vi "ParamReader2.vi"(8 "error in (no error)":errorcluster, 10 "what kind of binary":i32, 11 "selected path":path caption="selected \"*.par\" path") -> (0 "error out":errorcluster, 2 "CodeString":string, 5 "Cluster":T1 {"AdcOffset" format="%#.6f"; "AdcScale" format="%#.6f"})   [LabVIEW 2014]
panel:
  out "slow ADC\nactiveChannels\nRange":string
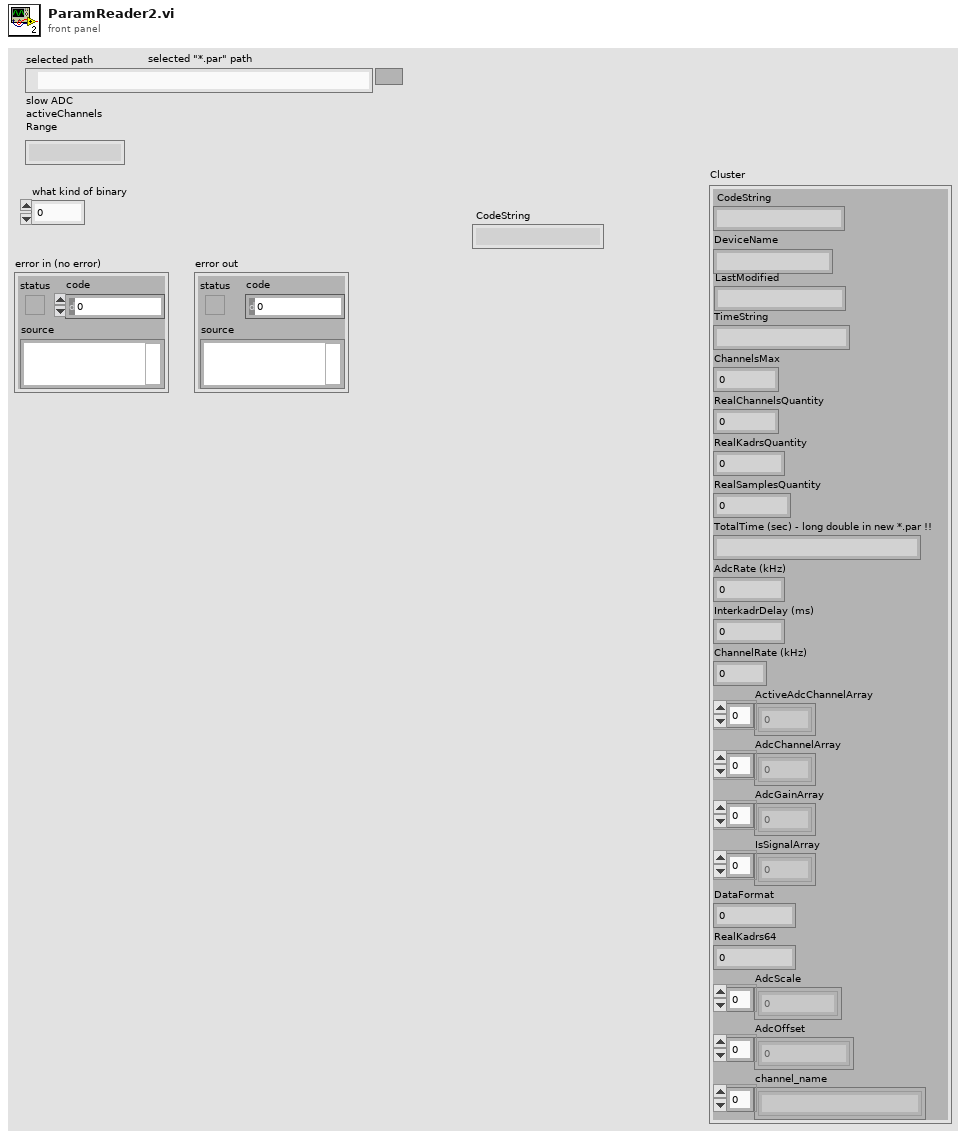
[diagram p1: front panel]
types:
  T1 = cluster{" CodeString":string, "DeviceName":string, "TimeString":string, "ChannelsMax":i16, "RealChannelsQuantity":i16, "RealKadrsQuantity":i64, "RealSamplesQuantity":i64, "TotalTime (sec) - long double in new *.par !!":string, "AdcRate (kHz)":dbl, "InterkadrDelay (ms)":dbl, "ChannelRate (kHz)":dbl, "ActiveAdcChannelArray":u32[], "AdcChannelArray":u8[], "AdcGainArray":u8[], "IsSignalArray":u8[], "DataFormat":i32, "RealKadrs64":i64, "AdcScale":dbl[], "AdcOffset":dbl[], "channel_name":string[], "LastModified":string}
  T2 = enum16{"open", "replace", "create", "open or create", "replace or create", "replace or create with confirmation"}
  T3 = enum16{"deny read/write", "deny write-only", "deny none"}
  T4 = enum16{"big-endian, network order", "native, host order", "little-endian"}
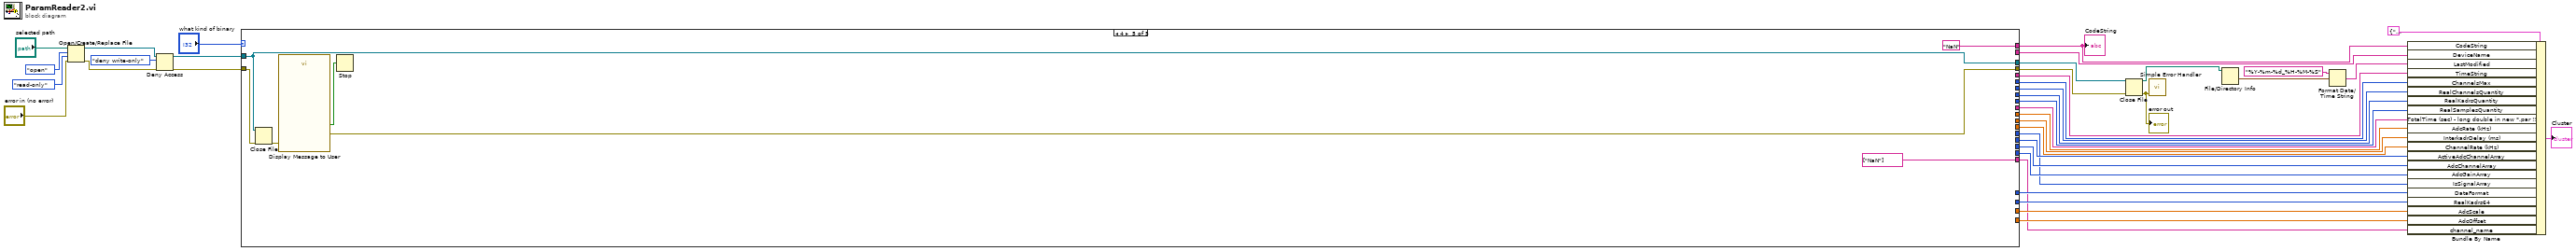
[diagram p0: block diagram]
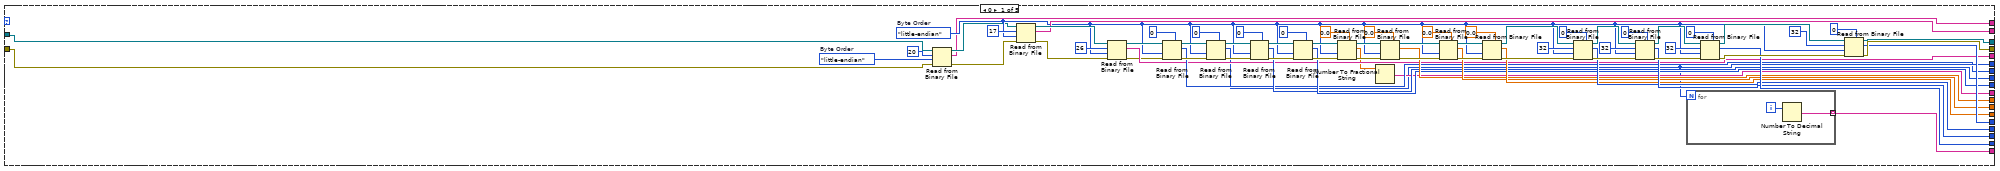
[diagram p2: hidden frame]
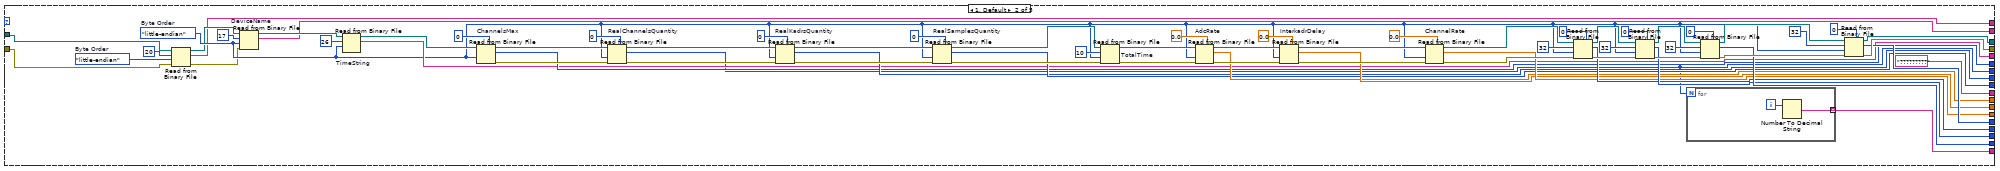
[diagram p3: hidden frame]
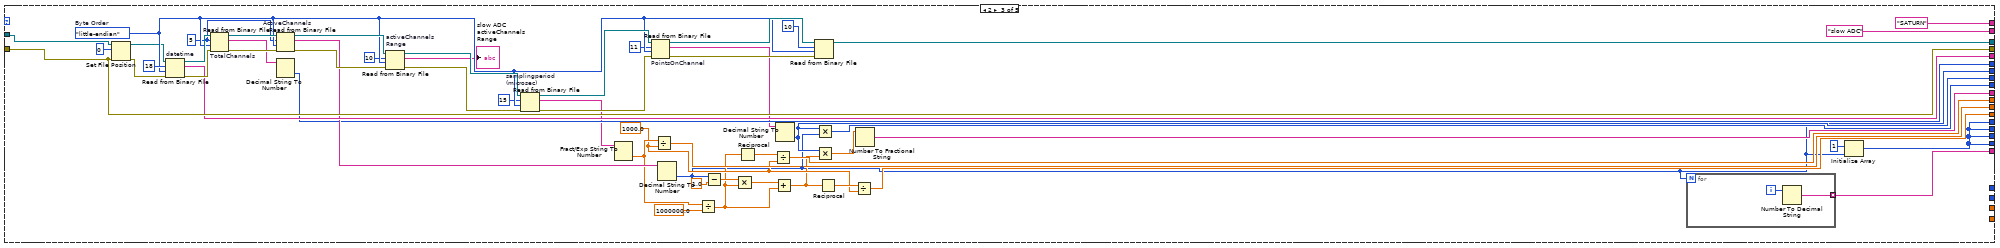
[diagram p4: hidden frame]
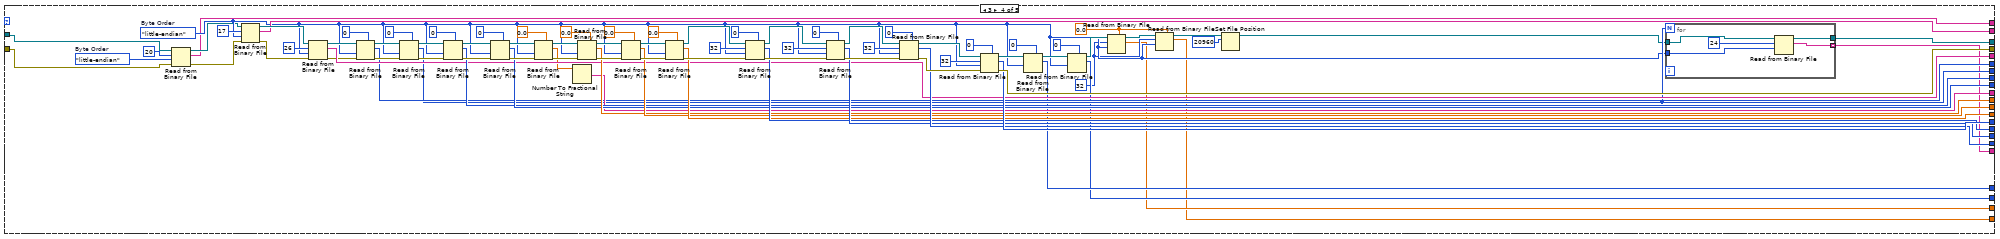
[diagram p5: hidden frame]
diagram:
  n1 = Open/Create/Replace File(file path (use dialog)="selected path", error in="error in (no error)", operation (0:open)=T2."open", access (0:read/write)=enum16{"read/write", "read-only", "write-only"}."read-only") -> (refnum out=w35:refnum<file>, error out=w34:errorcluster)  [unwired: 2 in, 1 out]
  n2 = Deny Access(4:w34, 6:T3."deny write-only" ("deny mode (0:deny read/write)"), 7:w35) -> (0:w9:errorcluster, 3:w8:refnum<file>)
  n3 = case shown="4" "what kind of binary" {
    tunnel: w8 -> [w44 w116 w220 w242 w330]
    tunnel: [w70 w136 w216 w283 w332] -> w38
    tunnel: w9 -> [w42 w114 w216 w240 w334]
    tunnel: [w69 w135 w213 w263 w330] -> w39
    tunnel: [w68 w134 w193 w282 _] -> w15
    tunnel: [w67 w133 w193 w281 _] -> w16
    tunnel: [w66 w132 w193 w280 _] -> w17
    tunnel: [w65 w131 w193 w279 _] -> w18
    tunnel: [w64 w130 w189 w278 _] -> w19
    tunnel: [w63 w129 w197 w277 _] -> w20
    tunnel: [w62 w128 w199 w276 _] -> w21
    tunnel: [w61 w127 w198 w275 _] -> w23
    tunnel: [w60 w126 w185 w274 _] -> w24
    tunnel: [w48 w119 w182 w261 _] -> w25
    tunnel: [w59 w125 w206 w262 _] -> w26
    tunnel: [w58 w124 w215 w273 _] -> w27
    tunnel: [w57 w123 "slow ADC" w272 _] -> w2
    tunnel: [w53 "?????????" w186 w268 _] -> w22
    tunnel: [w47 w120 w183 w260 string[] ["NaN"]] -> w10
    tunnel: [_ _ _ w250 _] -> w14
    tunnel: [_ _ _ w249 _] -> w13
    tunnel: [_ _ _ w246 _] -> w12
    tunnel: [_ _ _ w245 _] -> w11
    tunnel: [w40 w112 "SATURN" w238 "NaN"] -> w3
    frame 0 {
      w45 = T4."little-endian"  # Byte Order
      w49 = T4."little-endian"  # Byte Order
      n4 = Read from Binary File(8:w42, 9:w45, 10:20 ("count (1)"), 11:w44) -> (0:w41:errorcluster, 2:w40:string, 3:w43:refnum<file>)  [unwired: 2 in, 1 out]
      n5 = Read from Binary File(8:w41, 9:w49, 10:17 ("count (1)"), 11:w43) -> (0:w50:errorcluster, 2:w57:string, 3:w107:refnum<file>)  [unwired: 2 in, 1 out]
      n6 = Read from Binary File(8:w50, 9:w49, 10:26 ("count (1)"), 11:w107) -> (0:w51:errorcluster, 2:w58:string, 3:w105:refnum<file>)  [unwired: 2 in, 1 out]
      n7 = Read from Binary File(5:i16 0 ("count (1)"), 8:w51, 9:w49, 11:w105) -> (0:w92:errorcluster, 2:w59:i16, 3:w103:refnum<file>)  [unwired: 2 in, 1 out]
      n8 = Read from Binary File(5:i16 0 ("count (1)"), 8:w92, 9:w49, 11:w103) -> (0:w97:errorcluster, 2:w48:i16, 3:w96:refnum<file>)  [unwired: 2 in, 1 out]
      n9 = Read from Binary File(5:0 ("count (1)"), 8:w97, 9:w49, 11:w96) -> (0:w94:errorcluster, 2:w60:i32, 3:w95:refnum<file>)  [unwired: 2 in, 1 out]
      n10 = Read from Binary File(5:0 ("count (1)"), 8:w94, 9:w49, 11:w95) -> (0:w93:errorcluster, 2:w61:i32, 3:w55:refnum<file>)  [unwired: 2 in, 1 out]
      n11 = Read from Binary File(5:0.0 ("count (1)"), 8:w93, 9:w49, 11:w55) -> (0:w89:errorcluster, 2:w52:dbl, 3:w54:refnum<file>)  [unwired: 2 in, 1 out]
      n12 = Number To Fractional String(number=w52) -> (F-format string=w53:string)  [unwired: 3 in]
      n13 = Read from Binary File(5:sgl 0.0 ("count (1)"), 8:w89, 9:w49, 11:w54) -> (0:w88:errorcluster, 2:w62:sgl, 3:w91:refnum<file>)  [unwired: 2 in, 1 out]
      n14 = Read from Binary File(5:sgl 0.0 ("count (1)"), 8:w88, 9:w49, 11:w91) -> (0:w87:errorcluster, 2:w63:sgl, 3:w90:refnum<file>)  [unwired: 2 in, 1 out]
      n15 = Read from Binary File(5:sgl 0.0 ("count (1)"), 8:w87, 9:w49, 11:w90) -> (0:w83:errorcluster, 2:w64:sgl, 3:w84:refnum<file>)  [unwired: 2 in, 1 out]
      n16 = Read from Binary File(5:u8 0 ("count (1)"), 8:w83, 9:w49, 10:32 ("count (1)"), 11:w84) -> (0:w73:errorcluster, 2:w65:u8[], 3:w76:refnum<file>)  [unwired: 1 in, 1 out]
      n17 = Read from Binary File(5:u8 0 ("count (1)"), 8:w73, 9:w49, 10:32 ("count (1)"), 11:w76) -> (0:w72:errorcluster, 2:w66:u8[], 3:w75:refnum<file>)  [unwired: 1 in, 1 out]
      n18 = for {
        N: w48 -> [_]
        tunnel: [w111] -> w47 mode=indexing
        i -> [w110]
        n19 = Number To Decimal String(number=w110) -> (decimal integer string=w111:string)  [unwired: 1 in]
      }
      n20 = Read from Binary File(5:u8 0 ("count (1)"), 8:w72, 9:w49, 10:32 ("count (1)"), 11:w75) -> (0:w71:errorcluster, 2:w67:u8[], 3:w74:refnum<file>)  [unwired: 1 in, 1 out]
      n21 = Read from Binary File(5:u8 0 ("count (1)"), 8:w71, 9:w49, 10:32 ("count (1)"), 11:w74) -> (0:w70:errorcluster, 2:w68:u8[], 3:w69:refnum<file>)  [unwired: 1 in, 1 out]
    }
    frame 1, Default {
      w118 = T4."little-endian"  # Byte Order
      w121 = T4."little-endian"  # Byte Order
      n22 = Read from Binary File(8:w114, 9:w118, 10:20 ("count (1)"), 11:w116) -> (0:w113:errorcluster, 2:w112:string, 3:w115:refnum<file>)  [unwired: 2 in, 1 out]
      n23 = Read from Binary File "DeviceName"(8:w113, 9:w121, 10:17 ("count (1)"), 11:w115) -> (2:w123:string, 3:w176:refnum<file>)  [unwired: 2 in, 2 out]
      n24 = Read from Binary File "TimeString"(9:w121, 10:26 ("count (1)"), 11:w176) -> (2:w124:string, 3:w174:refnum<file>)  [unwired: 3 in, 2 out]
      n25 = Read from Binary File "ChannelsMax"(5:i16 0 ("count (1)"), 9:w121, 11:w174) -> (0:w159:errorcluster, 2:w125:i16, 3:w172:refnum<file>)  [unwired: 3 in, 1 out]
      n26 = Read from Binary File "RealChannelsQuantity"(5:i16 0 ("count (1)"), 8:w159, 9:w121, 11:w172) -> (0:w165:errorcluster, 2:w119:i16, 3:w164:refnum<file>)  [unwired: 2 in, 1 out]
      n27 = Read from Binary File "RealKadrsQuantity"(5:i64 0 ("count (1)"), 8:w165, 9:w121, 11:w164) -> (0:w161:errorcluster, 2:w126:i64, 3:w163:refnum<file>)  [unwired: 2 in, 1 out]
      n28 = Read from Binary File "RealSamplesQuantity"(5:i64 0 ("count (1)"), 8:w161, 9:w121, 11:w163) -> (0:w160:errorcluster, 2:w127:i64, 3:w162:refnum<file>)  [unwired: 2 in, 1 out]
      n29 = Read from Binary File "TotalTime"(8:w160, 9:w121, 10:10 ("count (1)"), 11:w162) -> (0:w155:errorcluster, 3:w158:refnum<file>)  [unwired: 2 in, 2 out]
      n30 = Read from Binary File "AdcRate"(5:0.0 ("count (1)"), 8:w155, 9:w121, 11:w158) -> (0:w154:errorcluster, 2:w128:dbl, 3:w157:refnum<file>)  [unwired: 2 in, 1 out]
      n31 = Read from Binary File "InterkadrDelay"(5:0.0 ("count (1)"), 8:w154, 9:w121, 11:w157) -> (0:w153:errorcluster, 2:w129:dbl, 3:w156:refnum<file>)  [unwired: 2 in, 1 out]
      n32 = Read from Binary File "ChannelRate"(5:0.0 ("count (1)"), 8:w153, 9:w121, 11:w156) -> (0:w149:errorcluster, 2:w130:dbl, 3:w150:refnum<file>)  [unwired: 2 in, 1 out]
      n33 = Read from Binary File(5:u32 0 ("count (1)"), 8:w149, 9:w121, 10:32 ("count (1)"), 11:w150) -> (0:w139:errorcluster, 2:w131:u32[], 3:w142:refnum<file>)  [unwired: 1 in, 1 out]
      n34 = Read from Binary File(5:u8 0 ("count (1)"), 8:w139, 9:w121, 10:32 ("count (1)"), 11:w142) -> (0:w138:errorcluster, 2:w132:u8[], 3:w141:refnum<file>)  [unwired: 1 in, 1 out]
      n35 = for {
        N: w119 -> [_]
        tunnel: [w180] -> w120 mode=indexing
        i -> [w179]
        n36 = Number To Decimal String(number=w179) -> (decimal integer string=w180:string)  [unwired: 1 in]
      }
      n37 = Read from Binary File(5:u8 0 ("count (1)"), 8:w138, 9:w121, 10:32 ("count (1)"), 11:w141) -> (0:w137:errorcluster, 2:w133:u8[], 3:w140:refnum<file>)  [unwired: 1 in, 1 out]
      n38 = Read from Binary File(5:u8 0 ("count (1)"), 8:w137, 9:w121, 10:32 ("count (1)"), 11:w140) -> (0:w136:errorcluster, 2:w134:u8[], 3:w135:refnum<file>)  [unwired: 1 in, 1 out]
    }
    frame 2 {
      w195 = 1000.0 ("y")
      w212 = 5 ("count (1)")
      w223 = T4."little-endian"  # Byte Order
      n39 = Set File Position(offset (in bytes) (0)=i64 0, refnum=w220, error in=w216) -> (refnum out=w218:refnum<file>, error out=w217:errorcluster)  [unwired: 1 in]
      n40 = Read from Binary File "datetime"(8:w217, 9:w223, 10:18 ("count (1)"), 11:w218) -> (0:w222:errorcluster, 2:w215:string, 3:w234:refnum<file>)  [unwired: 2 in, 1 out]
      n41 = Read from Binary File "TotalChannels"(8:w222, 9:w223, 10:w212, 11:w234) -> (0:w221:errorcluster, 2:w208:string, 3:w233:refnum<file>)  [unwired: 2 in, 1 out]
      n42 = Read from Binary File "ActiveChannels"(8:w221, 9:w223, 10:w212, 11:w233) -> (0:w224:errorcluster, 2:w207:string, 3:w232:refnum<file>)  [unwired: 2 in, 1 out]
      n43 = Decimal String To Number(string=w208) -> (number=w206:i32)  [unwired: 2 in, 1 out]
      n44 = Read from Binary File "activeChannels\nRange"(8:w224, 9:w223, 10:10 ("count (1)"), 11:w232) -> (0:w230:errorcluster, 2:→"slow ADC\nactiveChannels\nRange":string, 3:w229:refnum<file>)  [unwired: 2 in, 1 out]
      n45 = Read from Binary File "samplingperiod\n(microsec)"(8:w230, 9:w223, 10:i64 15 ("count (1)"), 11:w229) -> (0:w226:errorcluster, 2:w203:string, 3:w228:refnum<file>)  [unwired: 2 in, 1 out]
      n46 = Fract/Exp String To Number(string=w203) -> (number=w196:dbl)  [unwired: 3 in, 1 out]
      n47 = Read from Binary File "PointsOnChannel"(8:w226, 9:w223, 10:i64 11 ("count (1)"), 11:w228) -> (0:w225:errorcluster, 2:w205:string, 3:w227:refnum<file>)  [unwired: 2 in, 1 out]
      n48 = Divide(x=w196, y=w195) -> (x/y=w197:dbl)
      n49 = Decimal String To Number(string=w207) -> (number=w182:i32)  [unwired: 2 in, 1 out]
      n50 = Divide(x=w196, y=1000000.0) -> (x/y=w188:dbl)
      n51 = Subtract(x=w182, y=1.0) -> (x-y=w191:dbl)
      n52 = Multiply(x=w191, y=w188) -> (x*y=w190:dbl)
      n53 = Reciprocal(x=w188) -> (1/x=w200:dbl)
      n54 = Divide(x=w200, y=w195) -> (x/y=w199:dbl)
      n55 = Add(x=w190, y=w188) -> (x+y=w184:dbl)
      n56 = Decimal String To Number(string=w205) -> (number=w185:i32)  [unwired: 2 in, 1 out]
      n57 = Read from Binary File(8:w225, 9:w223, 10:10 ("count (1)"), 11:w227) -> (3:w213:refnum<file>)  [unwired: 2 in, 3 out]
      n58 = Multiply(x=w185, y=w182) -> (x*y=w198:i32)
      n59 = Multiply(x=w185, y=w184) -> (x*y=w187:dbl)
      n60 = Reciprocal(x=w184) -> (1/x=w202:dbl)
      n61 = Divide(x=w202, y=w195) -> (x/y=w189:dbl)
      n62 = Number To Fractional String(number=w187) -> (F-format string=w186:string)  [unwired: 3 in]
      n63 = for {
        N: w182 -> [_]
        tunnel: [w237] -> w183 mode=indexing
        i -> [w236]
        n64 = Number To Decimal String(number=w236) -> (decimal integer string=w237:string)  [unwired: 1 in]
      }
      n65 = Initialize Array(i8 1 ("element"), w182) -> (w193:i8[])
    }
    frame 3 {
      w244 = T4."little-endian"  # Byte Order
      w247 = 32 ("count (1)")
      w248 = 0.0 ("count (1)")
      w253 = T4."little-endian"  # Byte Order
      n66 = Read from Binary File(8:w240, 9:w244, 10:20 ("count (1)"), 11:w242) -> (0:w239:errorcluster, 2:w238:string, 3:w241:refnum<file>)  [unwired: 2 in, 1 out]
      n67 = Read from Binary File(8:w239, 9:w253, 10:17 ("count (1)"), 11:w241) -> (0:w265:errorcluster, 2:w272:string, 3:w320:refnum<file>)  [unwired: 2 in, 1 out]
      n68 = Read from Binary File(8:w265, 9:w253, 10:26 ("count (1)"), 11:w320) -> (0:w266:errorcluster, 2:w273:string, 3:w318:refnum<file>)  [unwired: 2 in, 1 out]
      n69 = Read from Binary File(5:i16 0 ("count (1)"), 8:w266, 9:w253, 11:w318) -> (0:w305:errorcluster, 2:w262:i16, 3:w316:refnum<file>)  [unwired: 2 in, 1 out]
      n70 = Read from Binary File(5:i16 0 ("count (1)"), 8:w305, 9:w253, 11:w316) -> (0:w310:errorcluster, 2:w261:i16, 3:w309:refnum<file>)  [unwired: 2 in, 1 out]
      n71 = Read from Binary File(5:0 ("count (1)"), 8:w310, 9:w253, 11:w309) -> (0:w307:errorcluster, 2:w274:i32, 3:w308:refnum<file>)  [unwired: 2 in, 1 out]
      n72 = Read from Binary File(5:0 ("count (1)"), 8:w307, 9:w253, 11:w308) -> (0:w306:errorcluster, 2:w275:i32, 3:w270:refnum<file>)  [unwired: 2 in, 1 out]
      n73 = Read from Binary File(5:0.0 ("count (1)"), 8:w306, 9:w253, 11:w270) -> (0:w302:errorcluster, 2:w267:dbl, 3:w269:refnum<file>)  [unwired: 2 in, 1 out]
      n74 = Number To Fractional String(number=w267) -> (F-format string=w268:string)  [unwired: 3 in]
      n75 = Read from Binary File(5:sgl 0.0 ("count (1)"), 8:w302, 9:w253, 11:w269) -> (0:w301:errorcluster, 2:w276:sgl, 3:w304:refnum<file>)  [unwired: 2 in, 1 out]
      n76 = Read from Binary File(5:sgl 0.0 ("count (1)"), 8:w301, 9:w253, 11:w304) -> (0:w300:errorcluster, 2:w277:sgl, 3:w303:refnum<file>)  [unwired: 2 in, 1 out]
      n77 = Read from Binary File(5:sgl 0.0 ("count (1)"), 8:w300, 9:w253, 11:w303) -> (0:w296:errorcluster, 2:w278:sgl, 3:w297:refnum<file>)  [unwired: 2 in, 1 out]
      n78 = Read from Binary File(5:u8 0 ("count (1)"), 8:w296, 9:w253, 10:32 ("count (1)"), 11:w297) -> (0:w286:errorcluster, 2:w279:u8[], 3:w289:refnum<file>)  [unwired: 1 in, 1 out]
      n79 = Read from Binary File(5:u8 0 ("count (1)"), 8:w286, 9:w253, 10:32 ("count (1)"), 11:w289) -> (0:w285:errorcluster, 2:w280:u8[], 3:w288:refnum<file>)  [unwired: 1 in, 1 out]
      n80 = Read from Binary File(5:u8 0 ("count (1)"), 8:w285, 9:w253, 10:32 ("count (1)"), 11:w288) -> (0:w284:errorcluster, 2:w281:u8[], 3:w287:refnum<file>)  [unwired: 1 in, 1 out]
      n81 = Read from Binary File(5:u8 0 ("count (1)"), 8:w284, 9:w253, 10:32 ("count (1)"), 11:w287) -> (0:w283:errorcluster, 2:w282:u8[], 3:w258:refnum<file>)  [unwired: 1 in, 1 out]
      n82 = Read from Binary File(5:0 ("count (1)"), 9:w253, 11:w258) -> (2:w250:i32, 3:w257:refnum<file>)  [unwired: 3 in, 2 out]
      n83 = Read from Binary File(5:i64 0 ("count (1)"), 9:w253, 11:w257) -> (2:w249:i64, 3:w256:refnum<file>)  [unwired: 3 in, 2 out]
      n84 = Read from Binary File(5:w248, 9:w253, 10:w247, 11:w256) -> (2:w246:dbl[], 3:w255:refnum<file>)  [unwired: 2 in, 2 out]
      n85 = Read from Binary File(5:w248, 9:w253, 10:w247, 11:w255) -> (2:w245:dbl[], 3:w254:refnum<file>)  [unwired: 2 in, 2 out]
      n86 = Set File Position(offset (in bytes) (0)=i64 20960, refnum=w254) -> (refnum out=w259:refnum<file>)  [unwired: 2 in, 1 out]
      n87 = for {
        N: w261 -> [_]
        tunnel: w253 -> [w325]
        tunnel: w259 -> [w327]
        tunnel: [w326] -> w263
        tunnel: [w324] -> w260 mode=indexing
        n88 = Read from Binary File(9:w325, 10:24 ("count (1)"), 11:w327) -> (2:w324:string, 3:w326:refnum<file>)  [unwired: 3 in, 2 out]
      }
    }
    frame 4 {
      n89 = Close File(refnum=w330, error in=w334) -> (error out=w333:errorcluster)  [unwired: 1 out]
      n90 = call "Display Message to User"("error in (no error)"=w333) -> ("error out"=w332:errorcluster, "OK"=w331:bool)  [unwired: 9 in]
      n91 = Stop(stop? (T)=w331) -> ()
    }
  }
  "CodeString" <- w3
  n92 = Close File(refnum=w39, error in=w38) -> (path=w6:path, error out=w32:errorcluster)
  "error out" <- w32
  n93 = call <vilib>:"Simple Error Handler.vi"("error in (no error)"=w32) -> ()  [unwired: 4 in, 5 out]
  n94 = File/Directory Info(path=w6) -> (last mod=w7:timestamp)  [unwired: 1 in, 6 out]
  n95 = Format Date/Time String(time format string (%c)="%Y-%m-%d_%H-%M-%S", seconds (now)=w7) -> (date/time string=w1:string)  [unwired: 1 in]
  n96 = Bundle By Name(cluster=T1 {" CodeString"="3571090,7859525  \u0000\u0000\u0000", "DeviceName"="E2010\u0000\u0000\u0000\u0000\u0000\u0000\u0000\u0000\u0000\u0000\u0000\u0000", "TimeString"="  02-10-2015 15:50:30\u0000\u0000\u0000\u0000\u0000", "ChannelsMax"=4, "RealChannelsQuantity"=4, "RealKadrsQuantity"=200000, "RealSamplesQuantity"=800000, "TotalTime (sec) - long double in new *.par !!"="0.080000", "AdcRate (kHz)"=2500.0, "InterkadrDelay (ms)"=9.999999747378752e-05, "ChannelRate (kHz)"=2500.0, "ActiveAdcChannelArray"=[1, 1, 1, 1, 0, 0, 0, 0, 0, 0, 0, 0, 0, 0, 0, 0, 0, 0, 0, 0, 0, 0, 0, 0, 0, 0, 0, 0, 0, 0, 0, 0], "AdcChannelArray"=[0, 1, 2, 3, 4, 5, 6, 7, 8, 9, 10, 11, 12, 13, 14, 15, 16, 17, 18, 19, 20, 21, 22, 23, 24, 25, 26, 27, 28, 29, 30, 31], "AdcGainArray"=[0, 0, 0, 0, 0, 0, 0, 0, 0, 0, 0, 0, 0, 0, 0, 0, 0, 0, 0, 0, 0, 0, 0, 0, 0, 0, 0, 0, 0, 0, 0, 0], "IsSignalArray"=[0, 0, 0, 0, 0, 0, 0, 0, 0, 0, 0, 0, 0, 0, 0, 0, 0, 0, 0, 0, 0, 0, 0, 0, 0, 0, 0, 0, 0, 0, 0, 0], "DataFormat"=3, "RealKadrs64"=200000, "AdcScale"=[1.1072238683700562, 1.1072763204574585, 1.107199788093567, 1.1072269678115845, 1.0556581020355225, 1.0552871227264404, 1.055243730545044, 1.0555833578109741, 1.0995646715164185, 1.0995484590530396, 1.0996085405349731, 1.099328875541687, 1.0, 1.0, 1.0, 1.0, 1.0, 1.0, 1.0, 1.0, 1.0, 1.0, 1.0, 1.0, 1.0, 1.0, 1.0, 1.0, 1.0, 1.0, 1.0, 1.0], "AdcOffset"=[-8.893548965454102, -8.418173789978027, -7.680645942687988, -9.022905349731445, -1.0585507154464722, 1.6397662162780762, 1.4740158319473267, -0.589760959148407, 81.70808410644531, 95.51783752441406, 84.60665893554688, 83.73567962646484, 0.0, 0.0, 0.0, 0.0, 0.0, 0.0, 0.0, 0.0, 0.0, 0.0, 0.0, 0.0, 0.0, 0.0, 0.0, 0.0, 0.0, 0.0, 0.0, 0.0], "channel_name"=["", "", "", "", "", "", "", "", "", "", "", "", "", "", "", "", "", "", "", "", "", "", "", "", "", "", "", "", "", "", "", "", "0"], "LastModified"=""} ("Cluster 2"), "CodeString"=w3, "DeviceName"=w2, "LastModified"=w1, "TimeString"=w27, "ChannelsMax"=w26, "RealChannelsQuantity"=w25, "RealKadrsQuantity"=w24, "RealSamplesQuantity"=w23, "TotalTime (sec) - long double in new *.par !!"=w22, "AdcRate (kHz)"=w21, "InterkadrDelay (ms)"=w20, "ChannelRate (kHz)"=w19, "ActiveAdcChannelArray"=w18, "AdcChannelArray"=w17, "AdcGainArray"=w16, "IsSignalArray"=w15, "DataFormat"=w14, "RealKadrs64"=w13, "AdcScale"=w12, "AdcOffset"=w11, "channel_name"=w10) -> (→"Cluster":T1)
